vi "SendToDataBase.vi"(6 "Put in?":bool, 7 "TableName":string, 8 "error in":errorcluster, 9 "BD_Op":T1 caption="Baza Danych" items=["Server", "Local DB"], 10 "Connection in":T4, 11 "tdms file in":refnum<k34>) -> (0 "error out":errorcluster, 1 "Modified?":bool, 2 "Connection out":T4, 3 "tdms file out":refnum<k34>, 4 "PropGraph":T2={"Raw Data"=[[0.0], [0.0234375], [0.9609375]], "Poperties"={"RMS values"=[], "Max"=[], "Min"=[], "A(8)"=[], "t"=0.0, "A(8) Axis"=0.0, "Aw"=[], "Ak 30min"=0.0, "Ak_axis"=0, "Spec"=[]}, "Power Spectrum / PSD"=[]})   [LabVIEW 2019]
uses:
  <vilib>/addons/database/Connection.llb/Conn ObjectReference.ctl
  Communication/TypeDef/#TypeDef_PropGraph.ctl
  Communication/TypeDef/#TypeDef_PropertiesToSave.ctl
  TypeDef/#TypeDef_DBMode.ctl
  Communication/TypeDef/#TypeDef_SetGet.ctl
  TypeDef/#TypeDef_DataToDatabase.ctl
  TypeDef/#TypeDef_FinalDataToDatabase.ctl
  Global_Freq.vi
  <vilib>/addons/database/_DB Variant To Data/Database Variant To Data.xnode
  <vilib>/addons/database/NI_Database_API.lvlib
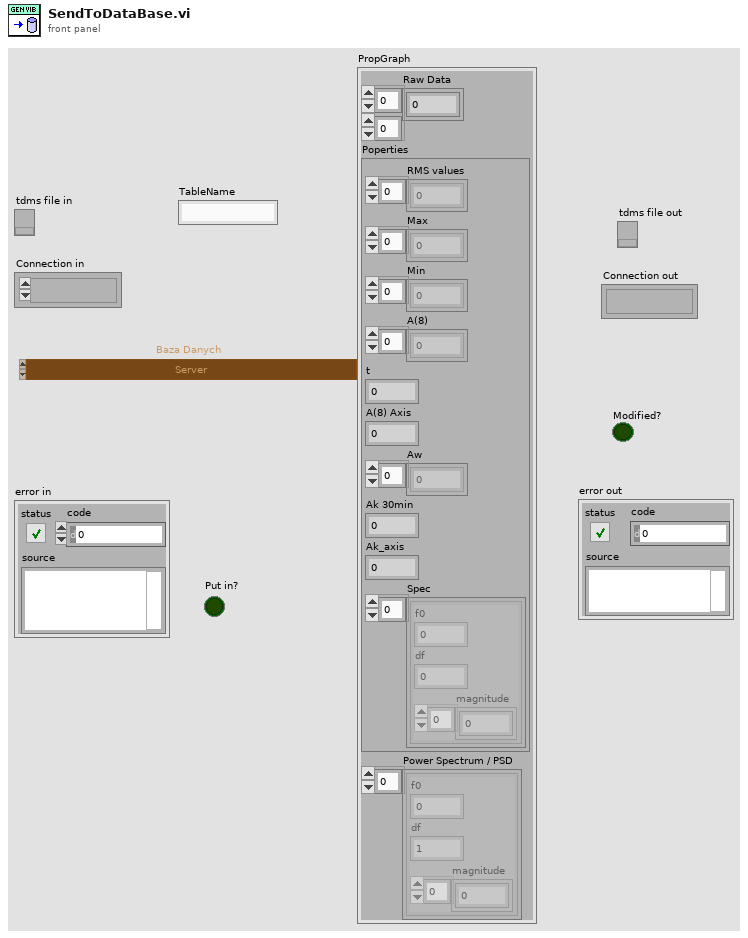
[diagram p1: front panel]
types:
  T1 = typedef "#TypeDef_DBMode.ctl" = u16
  T2 = typedef "#TypeDef_PropGraph.ctl" = cluster{"Raw Data":dbl[][], "Poperties":T3, "Power Spectrum / PSD":cluster{"f0":dbl, "df":dbl, "magnitude":dbl[]}[]}
  T3 = typedef "#TypeDef_PropertiesToSave.ctl" = cluster{"RMS values":dbl[], "Max":dbl[], "Min":dbl[], "A(8)":dbl[], "t":dbl, "A(8) Axis":dbl, "Aw":dbl[], "Ak 30min":dbl, "Ak_axis":i32, "Spec":cluster{"f0":dbl, "df":dbl, "magnitude":dbl[]}[]}
  T4 = typedef "NI_Database_API.lvlib/Conn ObjectReference.ctl" = refnum<k1>
  T5 = typedef "#TypeDef_SetGet.ctl" = enum16{"Set", "Get"}
  T6 = typedef "#TypeDef_DataToDatabase.ctl" = cluster{"RawDataX":dbl[], "RawDataY":dbl[], "RawDataZ":dbl[], "RMS values":dbl[], "Max":dbl[], "Min":dbl[], "Aw":dbl[], "A(8)":dbl[], "Ak Aray":dbl[], "t_A8Axis":dbl[]}
  T7 = typedef "#TypeDef_FinalDataToDatabase.ctl" = cluster{"A8":dbl[], "Ak Aray":dbl[]}
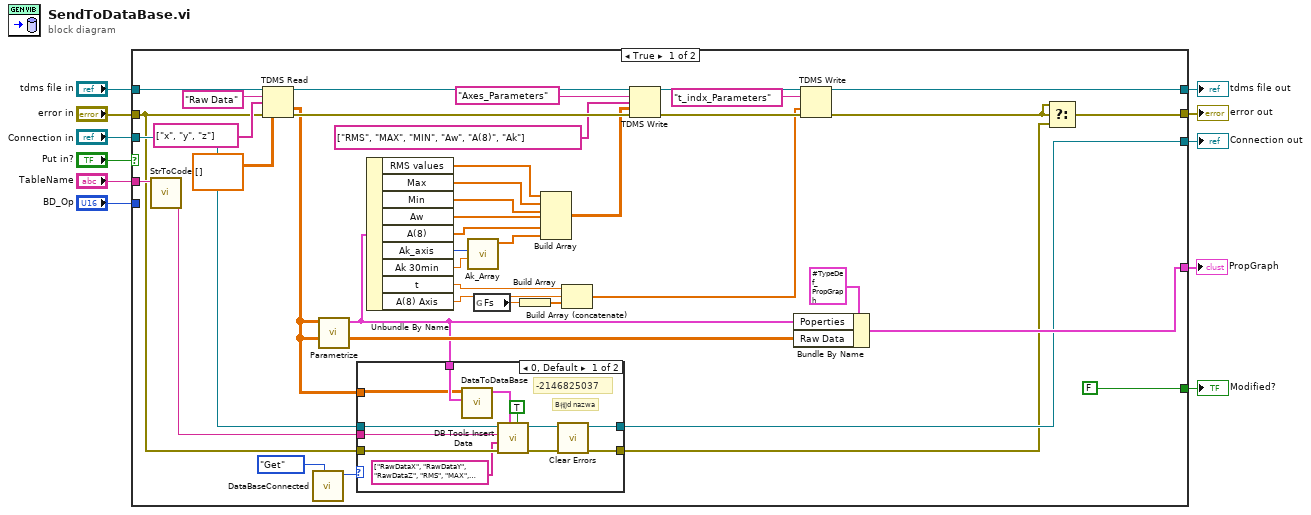
[diagram p0: block diagram]
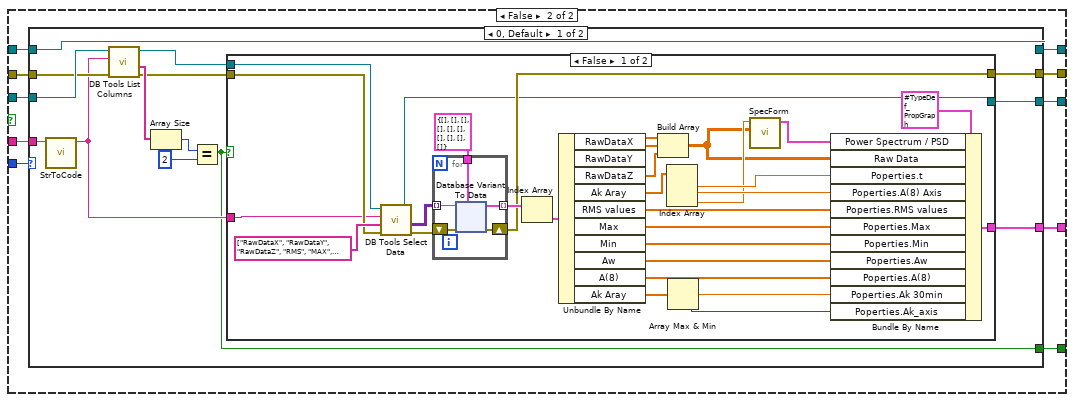
[diagram p3: hidden frame]
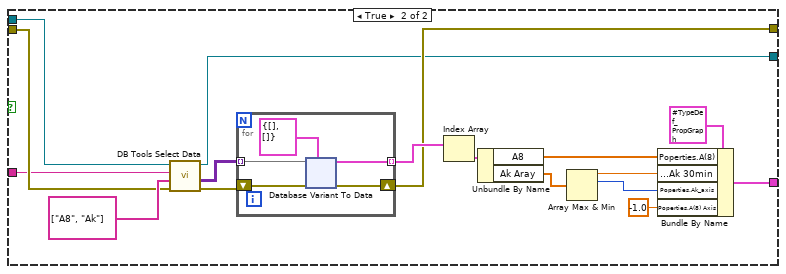
[diagram p4: hidden frame]
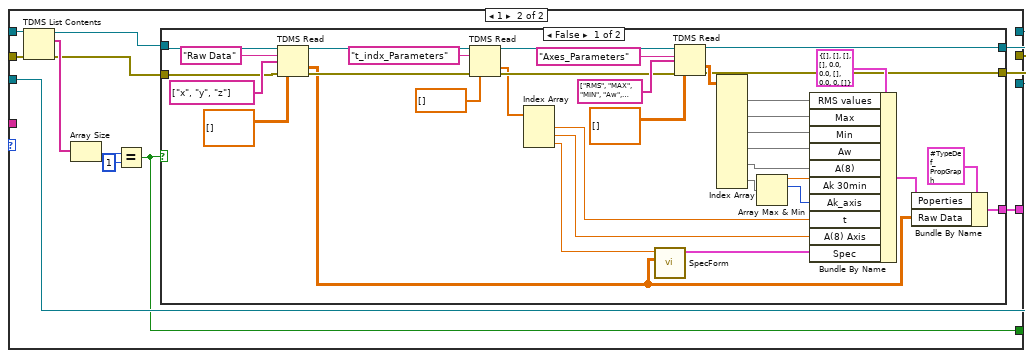
[diagram p5: hidden frame]
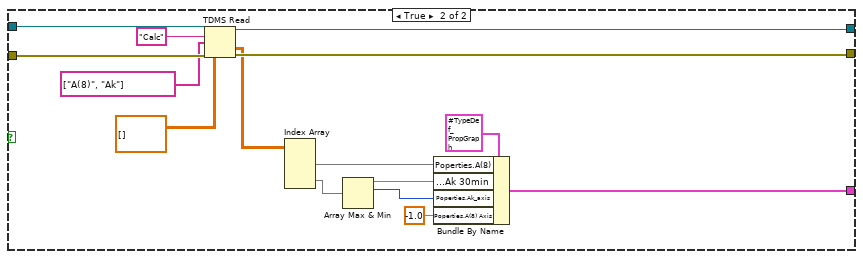
[diagram p6: hidden frame]
diagram:
  n1 = case shown="True" "Put in?" {
    tunnel: "error in" -> [w16 w71]
    tunnel: "tdms file in" -> [w15 w72]
    tunnel: [w49 w69] -> w3
    tunnel: "TableName" -> [w21 w74]
    tunnel: "Connection in" -> [w51 w75]
    tunnel: [w50 w67] -> w5
    tunnel: [w52 w70] -> w4
    tunnel: [w22 w68] -> w2
    tunnel: "BD_Op" -> [_ w73]
    tunnel: [FALSE w66] -> w1
    frame True {
      n2 = call "StrToCode.vi"("Name in"=w21) -> ("Name out"=w20:string)  [unwired: 10 in]
      n3 = TDMS Read(0:w15, 5:"Raw Data" ("group name in (Untitled)"), 7:string[] ["x", "y", "z"] ("channel name(s) in (Untitled)"), 11:w16, 12:dbl[][] [] ("RawData")) -> (4:w48:refnum<k34>, 10:w25:dbl[][], 15:w46:errorcluster)  [unwired: 3 in, 3 out]
      n4 = call "DataBaseConnected.vi"("Get/Set"=#TypeDef_SetGet."Get") -> ("BD out"=w18:T1)  [unwired: 10 in]
      n5 = call "Parametrize.vi"("Raw Data"=w25) -> ("Poperties"=w14:T3)  [unwired: 10 in]
      n6 = case shown="0, Default" w18 {
        tunnel: w51 -> [w63 w64]
        tunnel: [w62 w64] -> w50
        tunnel: w16 -> [w61 w65]
        tunnel: w14 -> [w58 _]
        tunnel: w25 -> [w57 _]
        tunnel: [w53 w65] -> w23
        tunnel: w20 -> [w55 _]
        frame 0, Default {
          # "B彻d nazwa"
          # "-2146825037"
          n7 = call "DataToDataBase.vi"("Poperties"=w58, "RawData"=w57) -> ("DataToDataBase"=w60:T6)  [unwired: 9 in]
          n8 = call <vilib>:"DB Tools Insert Data.vi"("create table? (F)"=TRUE, "data"=w60, "error in (no error)"=w61, "columns"=string[] ["RawDataX", "RawDataY", "RawDataZ", "RMS", "MAX", "MIN", "Aw", "A8", "Ak", "t_A8Axis"], "table"=w55, "connection reference"=w63) -> ("error out"=w54:errorcluster, "connection reference out"=w62:T4)  [unwired: 4 in]
          n9 = call <vilib>:"Clear Errors.vi"("error in (no error)"=w54) -> ("error out"=w53:errorcluster)  [unwired: 5 in, 1 out]
        }
        frame 1 {
        }
      }
      n10 = Unbundle By Name(w14) -> ("RMS values"=w34:dbl[], "Max"=w35:dbl[], "Min"=w36:dbl[], "Aw"=w42:dbl[], "A(8)"=w41:dbl[], "Ak_axis"=w27:i32, "Ak 30min"=w26:dbl, "t"=w39:dbl, "A(8) Axis"=w38:dbl)
      n11 = call "Ak_Array.vi"("Ak 30min"=w26, "Ak_axis"=w27) -> ("Ak Aray"=w28:dbl[])  [unwired: 9 in]
      n12 = global read "Global_Freq.vi" "Fs"() -> (w13:dbl)
      n13 = Build Array(w13) -> (w12:dbl[])
      n14 = Build Array(w34, w35, w36, w42, w41, w28) -> (w40:dbl[][])
      n15 = Build Array (concatenate)(w39, w38, w12) -> (w37:dbl[])
      n16 = TDMS Write(0:w48, 5:"Axes_Parameters" ("group name in (Untitled)"), 7:string[] ["RMS", "MAX", "MIN", "Aw", "A(8)", "Ak"] ("channel name(s) in (Untitled)"), 9:w40, 11:w46) -> (4:w47:refnum<k34>, 15:w45:errorcluster)  [unwired: 1 in, 2 out]
      n17 = Bundle By Name(cluster=T2 {"Raw Data"=[[0.0], [0.0234375], [0.9609375]], "Poperties"={"RMS values"=[], "Max"=[], "Min"=[], "A(8)"=[], "t"=0.0, "A(8) Axis"=0.0, "Aw"=[], "Ak 30min"=0.0, "Ak_axis"=0, "Spec"=[]}, "Power Spectrum / PSD"=[]} ("PropGraph"), "Poperties"=w14, "Raw Data"=w25) -> (w52:T2)
      n18 = TDMS Write(0:w47, 5:"t_indx_Parameters" ("group name in (Untitled)"), 9:w37, 11:w45) -> (4:w22:refnum<k34>, 15:w24:errorcluster)  [unwired: 2 in, 2 out]
      n19 = Select(t=w24, s=w24, f=w23) -> (s? t:f=w49:errorcluster)
    }
    frame False {
      n20 = case shown="0, Default" w73 {
        tunnel: w75 -> [w89 w564]
        tunnel: w74 -> [w78 _]
        tunnel: w72 -> [w80 w571]
        tunnel: w71 -> [w88 w570]
        tunnel: [w82 w567] -> w70
        tunnel: [w81 w566] -> w69
        tunnel: [w80 w565] -> w68
        tunnel: [w79 w564] -> w67
        tunnel: [w76 w563] -> w66
        frame 0, Default {
          n21 = call "StrToCode.vi"("Name in"=w78) -> ("Name out"=w77:string)  [unwired: 10 in]
          n22 = call <vilib>:"DB Tools List Columns.vi"("error in (no error)"=w88, "table"=w77, "connection reference"=w89) -> ("error out"=w84:errorcluster, "columns"=w87:string[], "connection reference out"=w83:T4)  [unwired: 1 in, 1 out]
          n23 = Array Size(array=w87) -> (size(s)=w86:i32)
          n24 = Equal?(x=w86, y=2) -> (x = y?=w76:bool)
          n25 = case shown="False" w76 {
            tunnel: w84 -> [w101 w474]
            tunnel: w83 -> [w100 w473]
            tunnel: w77 -> [w99 w472]
            tunnel: [w102 w471] -> w82
            tunnel: [w98 w470] -> w81
            tunnel: [w97 w469] -> w79
            frame False {
              n26 = call <vilib>:"DB Tools Select Data.vi"("error in (no error)"=w101, "columns"=string[] ["RawDataX", "RawDataY", "RawDataZ", "RMS", "MAX", "MIN", "Aw", "A8", "Ak", "t_A8Axis"], "table"=w99, "connection reference"=w100) -> ("error out"=w105:errorcluster, "data"=w106:variant[][], "connection reference out"=w97:T4)  [unwired: 2 in]
              n27 = for {
                tunnel: [w124] -> w107 mode=indexing
                shift-right: [w122] -> w98
                shift-left: w105 -> [w123]
                tunnel: w106 -> [w121] mode=indexing
                tunnel: T6 {"RawDataX"=[], "RawDataY"=[], "RawDataZ"=[], "RMS values"=[], "Max"=[], "Min"=[], "Aw"=[], "A(8)"=[], "Ak Aray"=[], "t_A8Axis"=[]} ("DataToDataBase") -> [w120]
                n28 = xnode "Database Variant To Data"("database variant"=w121, "error in (no error)"=w123, "type"=w120) -> ("data"=w124:T6, "error out"=w122:errorcluster)
              }
              n29 = Index Array(array=w107) -> (element=w108:T6)  [unwired: 1 in]
              n30 = Unbundle By Name(w108) -> ("RawDataX"=w109:dbl[], "RawDataY"=w110:dbl[], "RawDataZ"=w111:dbl[], "Ak Aray"=w95:dbl[], "RMS values"=w112:dbl[], "Max"=w113:dbl[], "Min"=w114:dbl[], "Aw"=w115:dbl[], "A(8)"=w116:dbl[], "Ak Aray"=w117:dbl[])
              n31 = Build Array(w109, w110, w111) -> (w91:dbl[][])
              n32 = Index Array(array=w95) -> (element #1=w94:dbl, element #2=w93:dbl, element #3=w92:dbl)  [unwired: 3 in]
              n33 = Array Max & Min(array=w117) -> (max value=w118:dbl, max index (indices)=w119:i32)  [unwired: 2 out]
              n34 = call "SpecForm.vi"("Data"=w91, "Fs"=w92) -> ("Power Spectrum / PSD"=w90:cluster{"f0":dbl, "df":dbl, "magnitude":dbl[]}[])  [unwired: 9 in]
              n35 = Bundle By Name(cluster=T2 {"Raw Data"=[[0.0], [0.0234375], [0.9609375]], "Poperties"={"RMS values"=[], "Max"=[], "Min"=[], "A(8)"=[], "t"=0.0, "A(8) Axis"=0.0, "Aw"=[], "Ak 30min"=0.0, "Ak_axis"=0, "Spec"=[]}, "Power Spectrum / PSD"=[]} ("PropGraph"), "Power Spectrum / PSD"=w90, "Raw Data"=w91, "Poperties.t"=w94, "Poperties.A(8) Axis"=w93, "Poperties.RMS values"=w112, "Poperties.Max"=w113, "Poperties.Min"=w114, "Poperties.Aw"=w115, "Poperties.A(8)"=w116, "Poperties.Ak 30min"=w118, "Poperties.Ak_axis"=w119) -> (w102:T2)
            }
            frame True {
              n36 = call <vilib>:"DB Tools Select Data.vi"("error in (no error)"=w474, "columns"=string[] ["A8", "Ak"], "table"=w472, "connection reference"=w473) -> ("error out"=w478:errorcluster, "data"=w479:variant[][], "connection reference out"=w469:T4)  [unwired: 2 in]
              n37 = for {
                tunnel: [w490] -> w480 mode=indexing
                shift-right: [w488] -> w470
                shift-left: w478 -> [w489]
                tunnel: w479 -> [w487] mode=indexing
                n38 = xnode "Database Variant To Data"("database variant"=w487, "error in (no error)"=w489, "type"=T7 {"A8"=[], "Ak Aray"=[]}) -> ("data"=w490:T7, "error out"=w488:errorcluster)
              }
              n39 = Index Array(array=w480) -> (element=w481:T7)  [unwired: 1 in]
              n40 = Unbundle By Name(w481) -> ("A8"=w484:dbl[], "Ak Aray"=w485:dbl[])
              n41 = Array Max & Min(array=w485) -> (max value=w482:dbl, max index (indices)=w483:i32)  [unwired: 2 out]
              n42 = Bundle By Name(cluster=T2 {"Raw Data"=[[0.0], [0.0234375], [0.9609375]], "Poperties"={"RMS values"=[], "Max"=[], "Min"=[], "A(8)"=[], "t"=0.0, "A(8) Axis"=0.0, "Aw"=[], "Ak 30min"=0.0, "Ak_axis"=0, "Spec"=[]}, "Power Spectrum / PSD"=[]} ("PropGraph"), "Poperties.A(8)"=w484, "Poperties.Ak 30min"=w482, "Poperties.Ak_axis"=w483, "Poperties.A(8) Axis"=-1.0) -> (w471:T2)
            }
          }
        }
        frame 1 {
          n43 = TDMS List Contents(4:w570, 7:w571) -> (0:w569:errorcluster, 2:w574:string[], 3:w568:refnum<k34>)  [unwired: 1 in, 1 out]
          n44 = Array Size(array=w574) -> (size(s)=w573:i32)
          n45 = Equal?(x=w573, y=1) -> (x = y?=w563:bool)
          n46 = case shown="False" w563 {
            tunnel: w569 -> [w590 w623]
            tunnel: w568 -> [w589 w624]
            tunnel: [w591 w611] -> w567
            tunnel: [w587 w621] -> w566
            tunnel: [w588 w622] -> w565
            frame False {
              n47 = TDMS Read(0:w589, 5:"Raw Data" ("group name in (Untitled)"), 7:string[] ["x", "y", "z"] ("channel name(s) in (Untitled)"), 11:w590, 12:dbl[][] [] ("appended array")) -> (4:w584:refnum<k34>, 10:w575:dbl[][], 15:w583:errorcluster)  [unwired: 3 in, 3 out]
              n48 = TDMS Read(0:w584, 5:"t_indx_Parameters" ("group name in (Untitled)"), 11:w583, 12:dbl[] [] ("appended array")) -> (4:w582:refnum<k34>, 10:w580:dbl[], 15:w581:errorcluster)  [unwired: 4 in, 3 out]
              n49 = Index Array(array=w580) -> (element #1=w579:dbl, element #2=w578:dbl, element #3=w576:dbl)  [unwired: 3 in]
              n50 = call "SpecForm.vi"("Data"=w575, "Fs"=w576) -> ("Power Spectrum / PSD"=w577:cluster{"f0":dbl, "df":dbl, "magnitude":dbl[]}[])  [unwired: 9 in]
              n51 = TDMS Read(0:w582, 5:"Axes_Parameters" ("group name in (Untitled)"), 7:string[] ["RMS", "MAX", "MIN", "Aw", "A(8)", "Ak"] ("channel name(s) in (Untitled)"), 11:w581, 12:dbl[][] [] ("appended array")) -> (4:w588:refnum<k34>, 10:w600:dbl[][], 15:w587:errorcluster)  [unwired: 3 in, 3 out]
              n52 = Index Array(array=w600) -> (element #1=w601:dbl[], element #2=w602:dbl[], element #3=w603:dbl[], element #4=w604:dbl[], element #5=w605:dbl[], element #6=w607:dbl[])  [unwired: 12 in]
              n53 = Array Max & Min(array=w607) -> (max value=w608:dbl, max index (indices)=w609:i32)  [unwired: 2 out]
              n54 = Bundle By Name(cluster=T3 {"RMS values"=[], "Max"=[], "Min"=[], "A(8)"=[], "t"=0.0, "A(8) Axis"=0.0, "Aw"=[], "Ak 30min"=0.0, "Ak_axis"=0, "Spec"=[]} ("Poperties"), "RMS values"=w601, "Max"=w602, "Min"=w603, "Aw"=w604, "A(8)"=w605, "Ak 30min"=w608, "Ak_axis"=w609, "t"=w579, "A(8) Axis"=w578, "Spec"=w577) -> (w606:T3)
              n55 = Bundle By Name(cluster=T2 {"Raw Data"=[[0.0], [0.0234375], [0.9609375]], "Poperties"={"RMS values"=[], "Max"=[], "Min"=[], "A(8)"=[], "t"=0.0, "A(8) Axis"=0.0, "Aw"=[], "Ak 30min"=0.0, "Ak_axis"=0, "Spec"=[]}, "Power Spectrum / PSD"=[]} ("PropGraph"), "Poperties"=w606, "Raw Data"=w575) -> (w591:T2)
            }
            frame True {
              n56 = TDMS Read(0:w624, 5:"Calc" ("group name in"), 7:string[] ["A(8)", "Ak"] ("channel name(s) in (Untitled)"), 11:w623, 12:dbl[][] [] ("appended array")) -> (4:w622:refnum<k34>, 10:w613:dbl[][], 15:w621:errorcluster)  [unwired: 3 in, 3 out]
              n57 = Index Array(array=w613) -> (element #1=w612:dbl[], element #2=w610:dbl[])  [unwired: 4 in]
              n58 = Array Max & Min(array=w610) -> (max value=w619:dbl, max index (indices)=w620:i32)  [unwired: 2 out]
              n59 = Bundle By Name(cluster=T2 {"Raw Data"=[[0.0], [0.0234375], [0.9609375]], "Poperties"={"RMS values"=[], "Max"=[], "Min"=[], "A(8)"=[], "t"=0.0, "A(8) Axis"=0.0, "Aw"=[], "Ak 30min"=0.0, "Ak_axis"=0, "Spec"=[]}, "Power Spectrum / PSD"=[]} ("PropGraph"), "Poperties.A(8)"=w612, "Poperties.Ak 30min"=w619, "Poperties.Ak_axis"=w620, "Poperties.A(8) Axis"=-1.0) -> (w611:T2)
            }
          }
        }
      }
    }
  }
  "error out" <- w3
  "tdms file out" <- w2
  "Connection out" <- w5
  "PropGraph" <- w4
  "Modified?" <- w1
